vi "读取Name.vi"(8 "error in (no error)":errorcluster caption="错误输入（无错误）", 11 "animal输入":refnum<class "animal.lvclass">) -> (0 "error out":errorcluster caption="错误输出", 2 "Name":string, 3 "animal输出":refnum<class "animal.lvclass">)   [LabVIEW 2018, in "animal.lvclass"]
uses:
  animal.lvclass
  animal.lvclass/animal.ctl
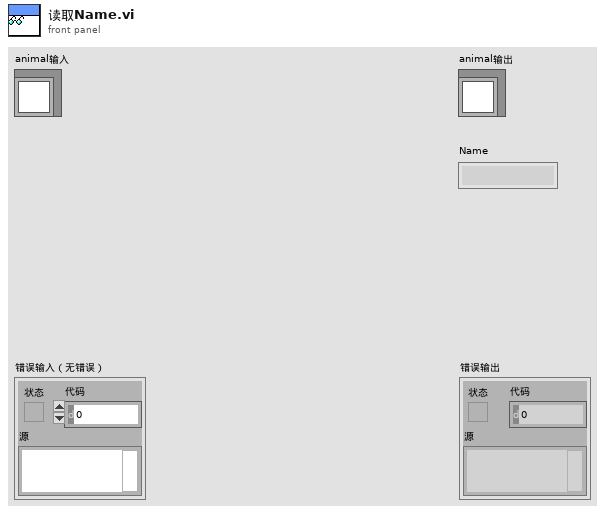
[diagram p1: front panel]
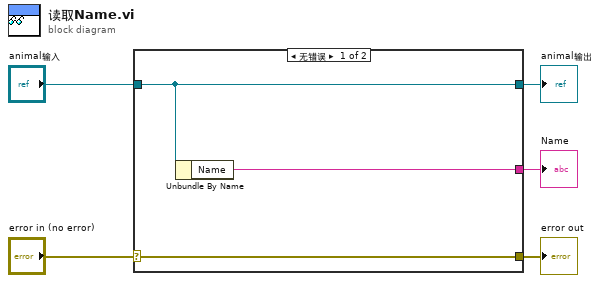
[diagram p0: block diagram]
diagram:
  n1 = case shown="无错误" "error in (no error)" {
    selector: "error in (no error)" -> [w8 w9]
    tunnel: [w8 w9] -> w4
    tunnel: [w7 w10] -> w2
    tunnel: "animal输入" -> [w7 w10]
    tunnel: [w6 _] -> w1
    frame No Error {
      n2 = Unbundle By Name(w7) -> ("Name"=w6:string)
    }
    frame Error {
    }
  }
  "error out" <- w4
  "animal输出" <- w2
  "Name" <- w1
